vi "GetText.vi"(8 "error in":errorcluster, 11 "PS Channel in":refnum<class "Power Supply Channel.lvclass">) -> (0 "error out":errorcluster, 1 "additional text":string, 2 "text":string, 3 "PS Channel out":refnum<class "Power Supply Channel.lvclass">, 4 "glyph":string)   [LabVIEW 2025, in "Power Supply.lvlib" / "Power Supply Channel.lvclass"]
doc: "Copyright 2017 National Instruments Corporation\n\nLicensed under the Apache License, Version 2.0 (the \"License\"); you may not use this file except in compliance with the License. You may obtain a copy of the License at http://www.apache.org/licenses/LICENSE-2.0\nUnless required by applicable law or agreed to in writing, software distributed under the License is distributed on an \"AS IS\" BASIS, WITHOUT WARRANTIES OR CONDITIONS OF ANY KIND, either express or implied. See the License for the specific language governing permissions and limitations under the License."
uses:
  Power Supply Channel.lvclass
  Power Supply Channel.lvclass/Power Supply Channel.ctl
  PS Channel configuration/Power Supply Channel configuration.lvclass
  C:/Users/Public/Documents/Sandia National Labs/TSS Plugin/Abstract Engine.lvlibp/Plugin/Abstract/Channel configuration/Channel configuration.lvclass
  Users/Public/Documents/Sandia National Labs/TSS Plugin/Abstract Engine.lvlibp/Plugin/Abstract/Channel configuration/Read Channel Setting.vi
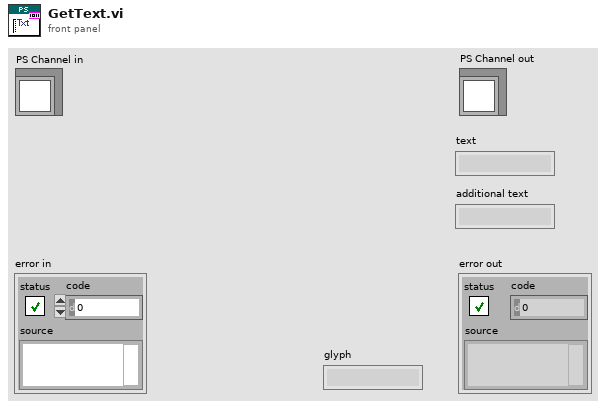
[diagram p1: front panel]
types:
  T1 = cluster{"Address":string, "SW Alias":string, "Description":string, "Enabled":bool, "Node Class":string}
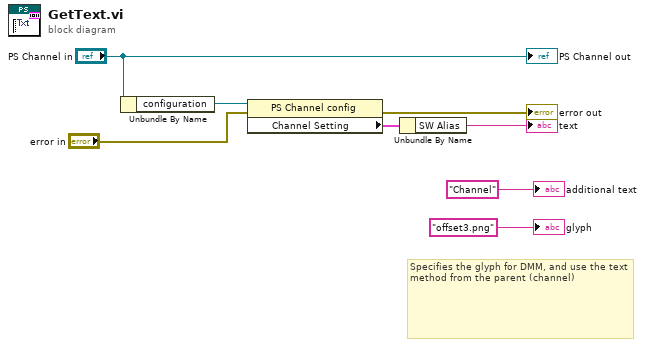
[diagram p0: block diagram]
diagram:
  # "Specifies the glyph for DMM, and use the text method from the parent (channel)"
  n1 = Unbundle By Name("PS Channel in") -> ("configuration"=w4:refnum<class "Power Supply Channel configuration.lvclass">)
  n2 = property class="PS Channel config"(reference=w4, error in="error in") -> (error out=→"error out":errorcluster, "Channel Setting"=w2:T1)  [unwired: 1 out]
  n3 = Unbundle By Name(w2) -> ("SW Alias"=→"text":string)
  "PS Channel out" <- "PS Channel in"
  "additional text" <- "Channel" ("additional text")
  "glyph" <- "offset3.png" ("glyph")
